vi "IECMemory.EnableCall.vi"(0 "i ref in":refnum<vi>, 1 "call process":string, 2 "call event":string, 3 "ms timeout (100)":i32=100, 5 "error in (no error)":errorcluster) -> (14 "i ref out":refnum<vi>, 17 "timed out":bool, 19 "error out":errorcluster)   [LabVIEW 2014, in "IECMemory.lvlib"]
doc: "This method can be used to check, if the PPG100 has finished to output its patterns. If that is the case, a call is sent to a specified process. How it works: \n\n1) it register the process and its event name that are specified by the caller\n2) Go to the poll state. In this state, the PPG100 checks its state via the periodic loop\n\nThe methods \"ppg handler\" and \"disable call\" are related to this method."
uses:
  IECMemory.lvlib
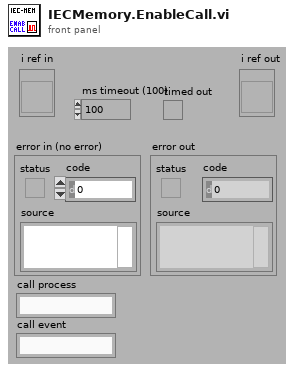
[diagram p1: front panel]
types:
  T1 = typedef "IECMemory.lvlib/IECMemory.i attribute.ctl" = cluster{"EndAddress":u32, "MemoryStatusBits":T2, "IEC Finished":bool, "Call Process":string, "Call Event":string}
  T2 = typedef "IECMemoryDriver.lvlib/Memory_Status.ctl" = bool[]
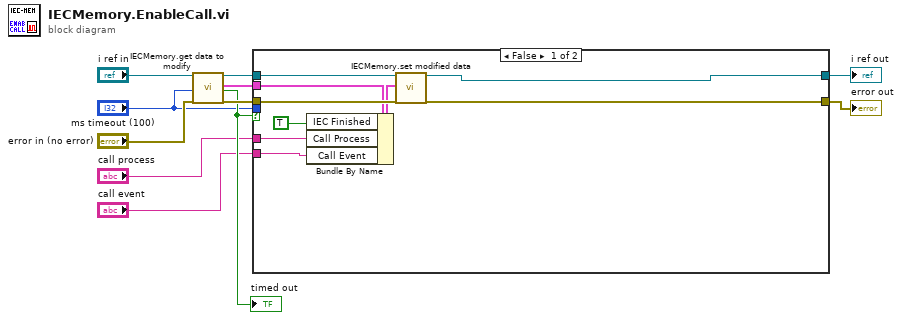
[diagram p0: block diagram]
diagram:
  n1 = call "IECMemory.get data to modify.vi"("i ref in"="i ref in", "ms timeout (10000)"="ms timeout (100)", "error in (no error)"="error in (no error)") -> ("i ref out"=w8:refnum<vi>, "i attribute"=w6:T1, "timed out"=w5:bool, "error out"=w7:errorcluster)  [unwired: 13 in]
  "timed out" <- w5
  n2 = case shown="False" w5 {
    tunnel: [w13 w21] -> w2
    tunnel: [w12 w22] -> w9
    tunnel: w8 -> [w20 w22]
    tunnel: w7 -> [w19 w21]
    tunnel: w6 -> [w17 _]
    tunnel: "call process" -> [w16 _]
    tunnel: "call event" -> [w15 _]
    tunnel: "ms timeout (100)" -> [_ _]
    frame False {
      n3 = Bundle By Name(cluster=w17, "IEC Finished"=TRUE ("PPG finished"), "Call Process"=w16, "Call Event"=w15) -> (w18:T1)
      n4 = call "IECMemory.set modified data.vi"("i ref in"=w20, "i attribute"=w18, "error in (no error)"=w19) -> ("i ref out"=w12:refnum<vi>, "error out"=w13:errorcluster)  [unwired: 15 in]
    }
    frame True {
    }
  }
  "error out" <- w2
  "i ref out" <- w9
